vi "Controller Configuration Loop.vi"(7 "Sync Objects":T2, 8 "error in (no error)":errorcluster, 11 "FOFB Configuration":T5={"FOFB Parameters"={"Network"={"FOFB Controller IP"="", "LNLS Control Network IP"="", "LNLS Control Network Power Supplies TCP Port"=0, "LNLS Control Network FOFB Configuration TCP Port"=0, "LNLS Control Network BPMs TCP Port"=0, "Monitoring Data TCP Port"=0, "Fast Archiver TCP Port"=0, "Fast Command TCP Port"=0, "TCP Listening Timeout"=0}, "Fast Acquisition"={"Sampling Period"=0, "Data Buffer Size"=0, "Monitoring Period"=0}, "Acquisition Network"=[], "Actuation Network"=[]}, "Number of Acquisition Chassis"=0, "Number of Actuation Chassis"=0, "Number of BPM Readings"=0, "BPM Reading Names"=[], "Selected BPM Readings"=[0, 1, 2, 3, 4, 5, 6, 7, 8, 9, 10, 11, 12, 13, 14, 15, 16, 17, 18, 19, 20, 21, 22, 23, 24, 25, 26, 27, 28, 29, 30, 31, 32, 33, 34, 35, 36, 37, 38, 39, 40, 41, 42, 43, 44, 45, 46, 47, 48, 49], "Number of Correctors"=0, "Corrector Names"=[], "Selected Correctors"=[0, 1, 2, 3, 4, 5, 6, 7, 8, 9, 10, 11, 12, 13, 14, 15, 16, 17, 18, 19, 20, 21, 22, 23, 24, 25, 26, 27, 28, 29, 30, 31, 32, 33, 34, 35, 36, 37, 38, 39, 40, 41, 42, 43, 44, 45, 46, 47, 48, 49], "Response Matrix"=[], "Reference Orbit"=[], "Correction Matrix"=[], "FPGA Filter Sets"=[], "Acquisition Chassis Names"=[], "Actuation Chassis Names"=[], "Acquisition Variables"=[], "Actuation Variables"=[], "PS Matrix Mapping"=[], "Inverse PS Matrix Mapping"=[], "BPM Matrix Mapping"=[], "Inverse BPM Matrix Mapping"=[], "BPM Planes"=[], "Corrector Planes"=[]}) -> (0 "error out":errorcluster)   [LabVIEW 2011, in "Controller VIs.lvlib"]
uses:
  Controller VIs.lvlib
  Types Definitions/Type FOFB Configuration.ctl
  Types Definitions/Type FOFB Parameters.ctl
  Types Definitions/Type Network Configuration.ctl
  Types Definitions/Type FA Configuration.ctl
  Types Definitions/Type Acquisition Network Configuration.ctl
  Types Definitions/Type Actuation Network Configuration.ctl
  Types Definitions/Type Synchronization Objects.ctl
  Types Definitions/Type Blocking Synchronization Objects.ctl
  Types Definitions/Type Monitoring Data.ctl
  Types Definitions/Type Operation Mode State.ctl
  Types Definitions/Type Diagnostics Data.ctl
  Types Definitions/Type CPU Loads Array.ctl
  Types Definitions/Type CPU Loads.ctl
  Types Definitions/Type Non-blocking Synchronization Objects.ctl
  Types Definitions/Type FOFB Variables.ctl
  Types Definitions/Type Actuation State.ctl
  <vilib>/Platform/TimedLoop/XDataNode/timing_clust.ctl
  <vilib>/Platform/TimedLoop/XDataNode/nitl_modes.ctl
  <vilib>/Platform/TimedLoop/XDataNode/wakeup.ctl
  Controller Global Variables/LNLS Control FOFB Configuration In.vi
  XML VIs/XML Get Actuation Chassis.vi
  XML VIs/XML Get Acquisition Chassis.vi
  <vilib>/Utility/libraryn.llb/Get File Extension.vi
  File VIs/File Read Matrix.vi
  Controller Orbit Correction Matrix Calculation.vi
  File VIs/File Write Matrix.vi
  File VIs/File Read Orbit.vi
  <vilib>/Utility/file.llb/Read From Spreadsheet File.vi
  <vilib>/Utility/file.llb/Read From Spreadsheet File (DBL).vi
  <vilib>/Platform/TimedLoop/XDataNode/XDataNode.xnode
  <vilib>/Platform/TimedLoop/XDataNode/XDNodeRunTimeDep.lvlib
  XML VIs.lvlib
  Controller Global Variables.lvlib
  Type Definitions.lvlib
panel:
  in  "FOFB Variables":T1
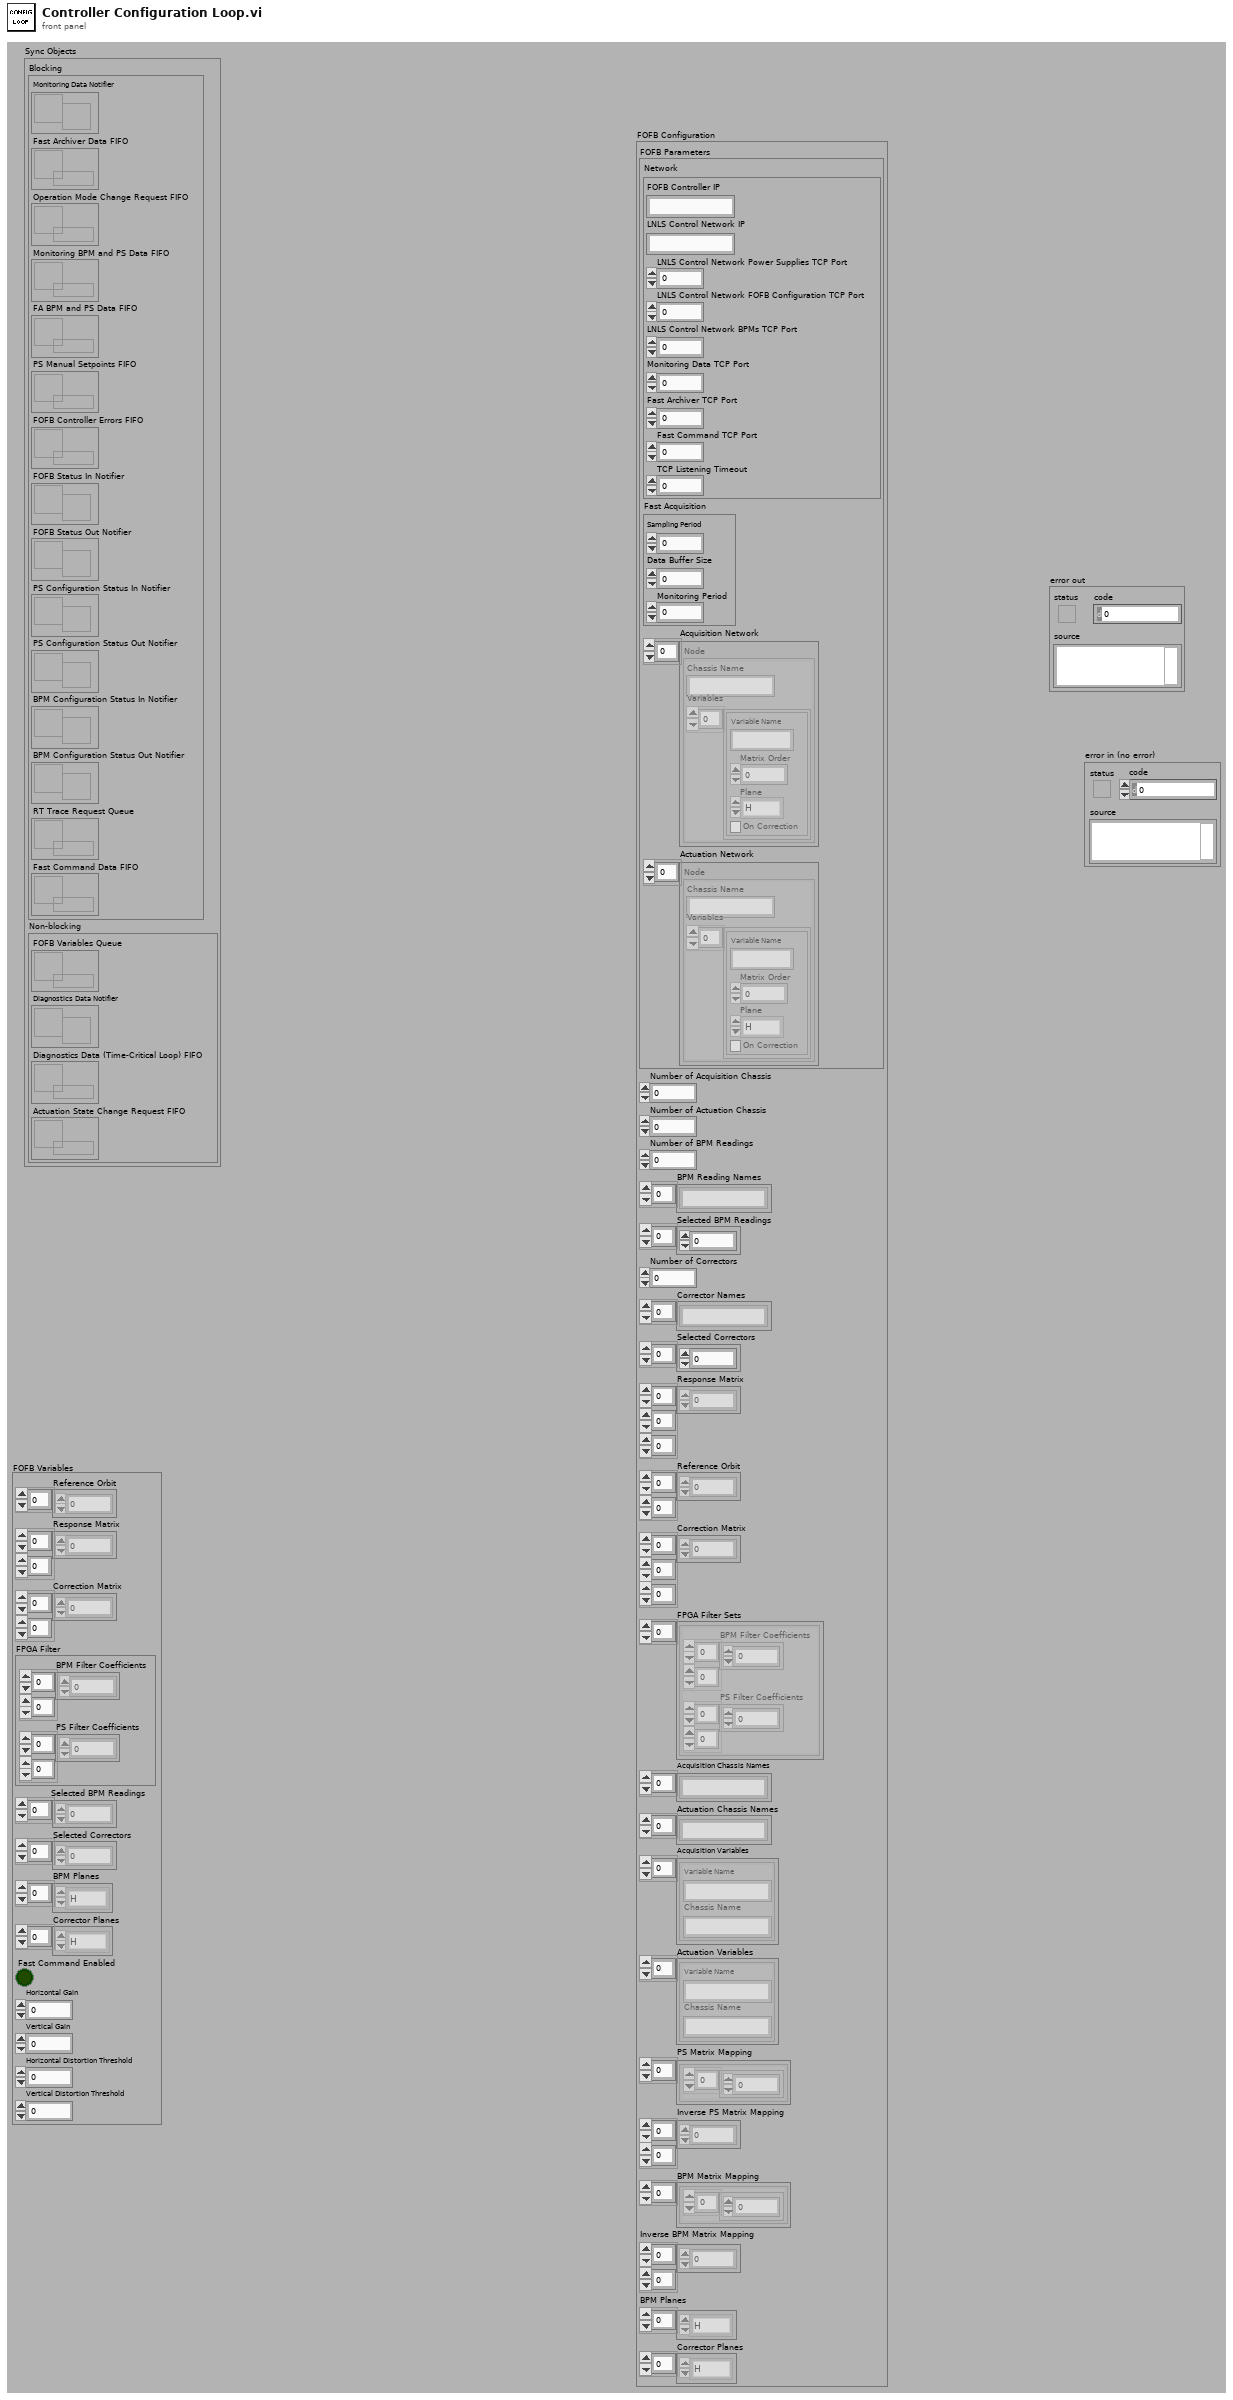
[diagram p1: front panel]
types:
  T1 = typedef "Type Definitions.lvlib/Type FOFB Variables.ctl" = cluster{"Reference Orbit":dbl[], "Response Matrix":dbl[][], "Correction Matrix":dbl[][], "FPGA Filter":cluster{"BPM Filter Coefficients":dbl[][], "PS Filter Coefficients":dbl[][]}, "Selected BPM Readings":u32[], "Selected Correctors":u32[], "BPM Planes":enum8{"H", "V"}[], "Corrector Planes":enum8{"H", "V"}[], "Fast Command Enabled":bool, "Horizontal Gain":dbl, "Vertical Gain":dbl, "Horizontal Distortion Threshold":dbl, "Vertical Distortion Threshold":dbl}
  T2 = typedef "Type Definitions.lvlib/Type Synchronization Objects.ctl" = cluster{"Blocking":T3, "Non-blocking":T4}
  T3 = typedef "Type Definitions.lvlib/Type Blocking Synchronization Objects.ctl" = cluster{"Monitoring Data Notifier":refnum<notifier>, "Fast Archiver Data FIFO":refnum<queue>, "Operation Mode Change Request FIFO":refnum<k33>, "Monitoring BPM and PS Data FIFO":refnum<k33>, "FA BPM and PS Data FIFO":refnum<k33>, "PS Manual Setpoints FIFO":refnum<k33>, "FOFB Controller Errors FIFO ":refnum<k33>, "FOFB Status In Notifier":refnum<notifier>, "FOFB Status Out Notifier":refnum<notifier>, "PS Configuration Status In Notifier":refnum<notifier>, "PS Configuration Status Out Notifier":refnum<notifier>, "BPM Configuration Status In Notifier":refnum<notifier>, "BPM Configuration Status Out Notifier":refnum<notifier>, "RT Trace Request Queue":refnum<queue>, "Fast Command Data FIFO":refnum<k33>}
  T4 = typedef "Type Definitions.lvlib/Type Non-blocking Synchronization Objects.ctl" = cluster{"FOFB Variables Queue":refnum<queue>, "Diagnostics Data Notifier":refnum<notifier>, "Diagnostics Data (Time-Critical Loop) FIFO":refnum<k33>, "Actuation State Change Request FIFO":refnum<k33>}
  T5 = typedef "Type Definitions.lvlib/Type FOFB Configuration.ctl" = cluster{"FOFB Parameters":T6, "Number of Acquisition Chassis":i32, "Number of Actuation Chassis":i32, "Number of BPM Readings":i32, "BPM Reading Names":string[], "Selected BPM Readings":u32[], "Number of Correctors":i32, "Corrector Names":string[], "Selected Correctors":u32[], "Response Matrix":dbl[][][], "Reference Orbit":dbl[][], "Correction Matrix":dbl[][][], "FPGA Filter Sets":cluster{"BPM Filter Coefficients":dbl[][], "PS Filter Coefficients":dbl[][]}[], "Acquisition Chassis Names":string[], "Actuation Chassis Names":string[], "Acquisition Variables":cluster{"Variable Name":string, "Chassis Name":string}[], "Actuation Variables":cluster{"Variable Name":string, "Chassis Name":string}[], "PS Matrix Mapping":cluster{u32[]}[], "Inverse PS Matrix Mapping":u32[][], "BPM Matrix Mapping":cluster{u32[]}[], "Inverse BPM Matrix Mapping":u32[][], "BPM Planes":enum8{"H", "V"}[], "Corrector Planes":enum8{"H", "V"}[]}
  T6 = typedef "Type Definitions.lvlib/Type FOFB Parameters.ctl" = cluster{"Network":T7, "Fast Acquisition":T8, "Acquisition Network":T9, "Actuation Network":T10}
  T7 = typedef "Type Definitions.lvlib/Type Network Configuration.ctl" = cluster{"FOFB Controller IP":string, "LNLS Control Network IP":string, "LNLS Control Network Power Supplies TCP Port":u16, "LNLS Control Network FOFB Configuration TCP Port":u16, "LNLS Control Network BPMs TCP Port":u16, "Monitoring Data TCP Port":u16, "Fast Archiver TCP Port":u16, "Fast Command TCP Port":u16, "TCP Listening Timeout":i32}
  T8 = typedef "Type Definitions.lvlib/Type FA Configuration.ctl" = cluster{"Sampling Period":u32, "Data Buffer Size":u32, "Monitoring Period":u32}
  T9 = typedef "Type Definitions.lvlib/Type Acquisition Network Configuration.ctl" = cluster{"Chassis Name":string, "Variables":cluster{"Variable Name":string, "Matrix Order":u32, "Plane":enum8{"H", "V"}, "On Correction":bool}[]}[]
  T10 = typedef "Type Definitions.lvlib/Type Actuation Network Configuration.ctl" = cluster{"Chassis Name":string, "Variables":cluster{"Variable Name":string, "Matrix Order":u32, "Plane":enum8{"H", "V"}, "On Correction":bool}[]}[]
  T11 = typedef "XDNodeRunTimeDep.lvlib/timing_clust.ctl" = cluster{"Expected End [f-1]":u64, "Actual End [f-1]":u64, "Finished Late? [f-1]":bool, "Expected End [i-1]":u64, "Actual End [i-1]":u64, "Finished Late? [i-1]":bool, "Expected Start [i]":u64, "Actual Start [i]":u64, "Expected Start [f]":u64, "Actual Start [f]":u64, "Source Name":string, "Structure Name":string, "Period":i64, "Deadline":i64, "Offset":i64, "Start":i64, "Priority":i32, "Timeout":i32, "Mode":T12, "Wakeup Reason":T13, "Error":errorcluster, "Source Type":string, "Secondary Source Type":string, "Global End Time":u64, "Global Start Time":u64, "Frame Duration":u64, "Iteration Duration":u64, "Assigned CPU":i32, "I/O Scan Engine Mode":u32}
  T12 = typedef "XDNodeRunTimeDep.lvlib/nitl_modes.ctl" = enum32{"No Change", "Process missed periods, maintain original phase", "Discard missed periods, maintain original phase", "Process missed periods, ignore original phase", "Discard missed periods, ignore original phase"}
  T13 = typedef "XDNodeRunTimeDep.lvlib/wakeup.ctl" = enum32{"Normal", "Aborted", "Asynchronous wakeup", "Timing source error", "Timed loop error", "Timeout"}
  T14 = typedef "Type Definitions.lvlib/Type Control FOFB Configuration In.ctl" = cluster{"Status":u16, "Operation Mode":T15, "Horizontal Gain":sgl, "Vertical Gain":sgl, "Selected Reference Orbit":i32, "Selected Correction Matrix":i32, "Selected FPGA Filters":i32, "Horizontal Distortion Threshold":sgl, "Vertical Distortion Threshold":sgl, "Fast Command Enabled":bool, "Update Reference Orbit":bool, "Update Contoller Configuration":bool}
  T15 = typedef "Type Definitions.lvlib/Type Operation Mode State.ctl" = enum8{"Idle Mode", "Manual Mode", "FOFB Mode"}
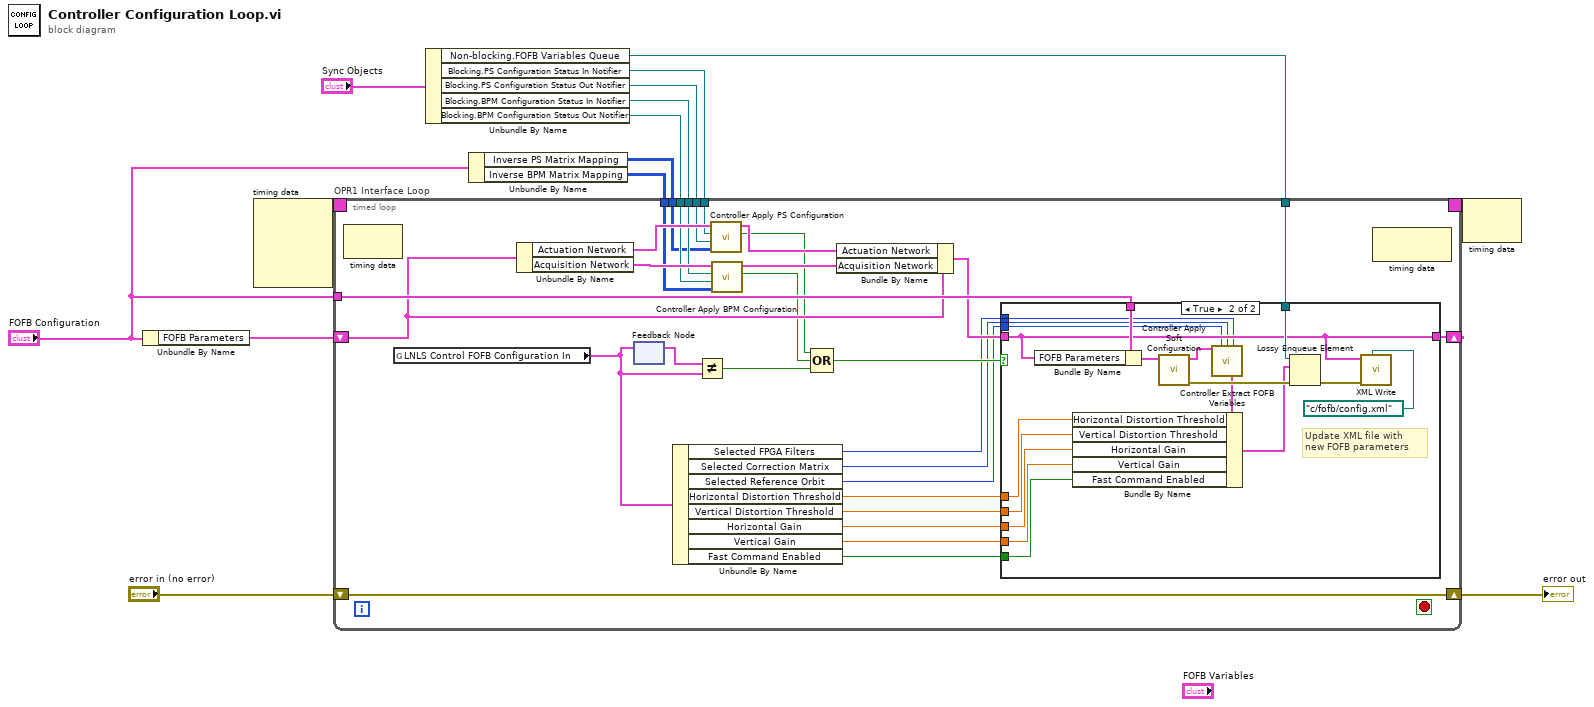
[diagram p0: block diagram]
diagram:
  n1 = Unbundle By Name("FOFB Configuration") -> ("FOFB Parameters"=w11:T6)
  n2 = node-c288() -> (w13:T11)  [unwired: 4 in]
  n3 = Unbundle By Name("Sync Objects") -> ("Non-blocking.FOFB Variables Queue"=w8:refnum<queue>, "Blocking.PS Configuration Status In Notifier"=w6:refnum<notifier>, "Blocking.PS Configuration Status Out Notifier"=w5:refnum<notifier>, "Blocking.BPM Configuration Status In Notifier"=w4:refnum<notifier>, "Blocking.BPM Configuration Status Out Notifier"=w3:refnum<notifier>)
  n4 = Unbundle By Name("FOFB Configuration") -> ("Inverse PS Matrix Mapping"=w2:u32[][], "Inverse BPM Matrix Mapping"=w1:u32[][])
  n5 = timed-loop "OPR1 Interface Loop" {
    timing: w13 -> [_]
    timing-out: [_] -> w12
    shift-right: [w42] -> _
    shift-left: w11 -> [w33]
    tunnel: w8 -> [w44]
    tunnel: "FOFB Configuration" -> [w43]
    shift-right: [w40] -> w10
    shift-left: "error in (no error)" -> [w40]
    tunnel: w6 -> [w30]
    tunnel: w5 -> [w29]
    tunnel: w4 -> [w28]
    tunnel: w3 -> [w27]
    tunnel: w2 -> [w26]
    tunnel: w1 -> [w25]
    stop <- _ stop-if-true
    n6 = node-c288() -> ()  [unwired: 1 in, 1 out]
    n7 = global read "LNLS Control FOFB Configuration In.vi" "LNLS Control FOFB Configuration In"() -> (w39:T14)
    n8 = Unbundle By Name(w33) -> ("Actuation Network"=w32:T10, "Acquisition Network"=w31:T9)
    n9 = feedback-in #1(w39) -> ()
    n10 = feedback #1() -> (w41:T14)  [unwired: 1 in]
    n11 = Unbundle By Name(w39) -> ("Selected FPGA Filters"=w15:i32, "Selected Correction Matrix"=w16:i32, "Selected Reference Orbit"=w17:i32, "Horizontal Distortion Threshold"=w34:sgl, "Vertical Distortion Threshold"=w35:sgl, "Horizontal Gain"=w36:sgl, "Vertical Gain"=w37:sgl, "Fast Command Enabled"=w38:bool)
    n12 = Not Equal?(x=w41, y=w39) -> (x != y?=w21:bool)
    n13 = call "Controller Apply PS Configuration.vi"("Inverse PS Matrix Mapping"=w26, "PS Configuration Status Out"=w29, "PS Configuration Status In"=w30, "Actuation Network In"=w32) -> ("Changed?"=w19:bool, "Actuation Network Out"=w24:T10)  [unwired: 6 in]
    n14 = call "Controller Apply BPM Configuration.vi"("Inverse BPM Matrix Mapping"=w25, "BPM Configuration Status Out"=w27, "BPM Configuration Status In"=w28, "Acquisition Network In"=w31) -> ("Changed?"=w18:bool, "Acquisition Network Out"=w23:T9)  [unwired: 6 in]
    n15 = Compound Arithmetic op=OR(w19, w18, w21) -> (w20:bool)
    n16 = Bundle By Name(cluster=w33, "Actuation Network"=w24, "Acquisition Network"=w23) -> (w22:T6)
    n17 = case shown="True" w20 {
      tunnel: w44 -> [_ w63]
      tunnel: w43 -> [_ w62]
      tunnel: w22 -> [w45 w57]
      tunnel: [w45 w57] -> w42
      tunnel: w38 -> [_ w53]
      tunnel: w37 -> [_ w52]
      tunnel: w36 -> [_ w51]
      tunnel: w15 -> [_ w50]
      tunnel: w16 -> [_ w49]
      tunnel: w17 -> [_ w48]
      tunnel: w35 -> [_ w47]
      tunnel: w34 -> [_ w46]
      frame False {
      }
      frame True {
        # "Update XML file with\nnew FOFB parameters"
        n18 = Bundle By Name(cluster=w62, "FOFB Parameters"=w57) -> (w56:T5)
        n19 = call "Controller Apply Soft Configuration.vi"("FOFB Configuration"=w56) -> ("error out"=w60:errorcluster, "FOFB Configuration"=w61:T5)  [unwired: 9 in]
        n20 = call "Controller Extract FOFB Variables.vi"("FOFB Configuration"=w61, "Selected Reference Orbit"=w48, "Selected Correction Matrix"=w49, "Selected FPGA Filters"=w50) -> ("FOFB Variables"=w55:T1)  [unwired: 10 in, 1 out]
        n21 = Bundle By Name(cluster=w55, "Horizontal Distortion Threshold"=w46, "Vertical Distortion Threshold"=w47, "Horizontal Gain"=w51, "Vertical Gain"=w52, "Fast Command Enabled"=w53) -> (w54:T1)
        n22 = Lossy Enqueue Element(queue=w63, element=w54, error in (no error)=w60) -> (error out=w59:errorcluster)  [unwired: 3 out]
        n23 = call "XML Write.vi"("XML File Path Write"=path "c:/fofb/config.xml" ("Configuration File Path"), "Error In"=w59, "FOFB Parameters"=w57) -> ()  [unwired: 7 in, 2 out]
      }
    }
    n24 = node-c288() -> ()  [unwired: 1 in, 1 out]
  }
  "error out" <- w10
  n25 = node-c288(w12) -> ()  [unwired: 1 out]
